vi "DMD_split_BMP.vi"(4 "error in (no error)":errorcluster, 5 "Packetlänge":i32=65535, 6 "Path":path, 7 "DMD in":refnum<class "DMD.lvclass">) -> (0 "error out":errorcluster, 1 "Packets":u8[][](array[numeric]) format="%x", 2 "Number of Packets":i16, 3 "DMD out":refnum<class "DMD.lvclass">)   [LabVIEW 2013, in "DMD.lvclass"]
uses:
  DMD.lvclass
panel:
  out "File-size":i32
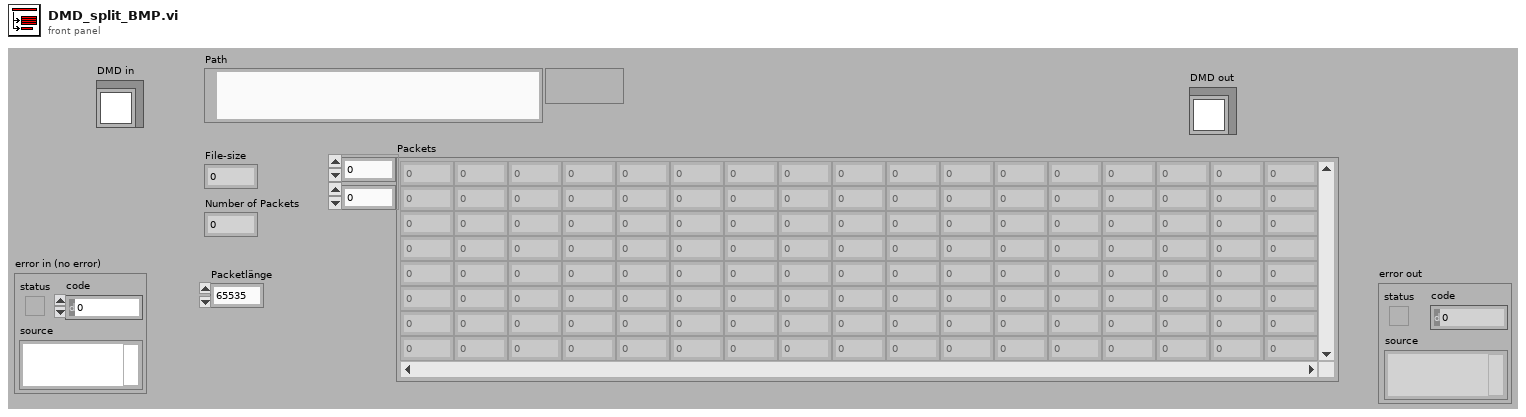
[diagram p1: front panel]
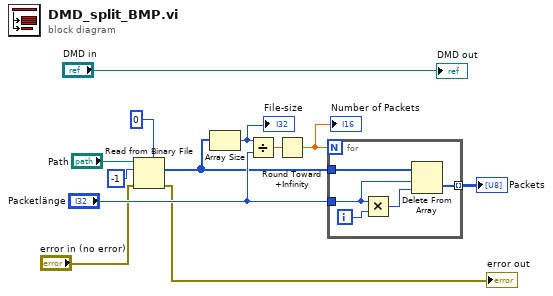
[diagram p0: block diagram]
diagram:
  n1 = Read from Binary File(5:u8 0, 8:"error in (no error)", 10:-1 ("count (1)"), 11:"Path") -> (0:→"error out":errorcluster, 2:w5:u8[])  [unwired: 2 in, 2 out]
  n2 = Array Size(array=w5) -> (size(s)=w10:i32)
  "File-size" <- w10
  n3 = Divide(x=w10, y="Packetlänge") -> (x/y=w12:dbl)
  n4 = Round Toward +Infinity(x=w12) -> (ceil(x): smallest int >= x=w11:dbl)
  "Number of Packets" <- w11
  n5 = for {
    N: w11 -> [_]
    tunnel: "Packetlänge" -> [w15]
    tunnel: w5 -> [w17]
    tunnel: [w13] -> w8 mode=indexing
    i -> [w16]
    n6 = Multiply(x=w15, y=w16) -> (x*y=w14:i32)
    n7 = Delete From Array(array=w17, length=w15, index=w14) -> (deleted portion=w13:u8[])  [unwired: 1 out]
  }
  "Packets" <- w8
  "DMD out" <- "DMD in"
